vi "TileFPWindows.vi"(5 "Tile Cols":i16=2, 7 "Tile Rows":i16=3, 8 "error in (no error)":errorcluster, 9 "Control Panel Bounds":T1, 10 "Monitor Bounds":T1, 11 "Number of channels":i32) -> (0 "error out":errorcluster, 1 "Not Enough Tiles":bool, 2 "Plot Bounds":T2(array[cluster]))   [LabVIEW 2015]
uses:
  <vilib>/Utility/miscctls.llb/LVRectTypeDef.ctl
panel:
  out "Numeric":i32=1
  out "Numeric 2":i32=1
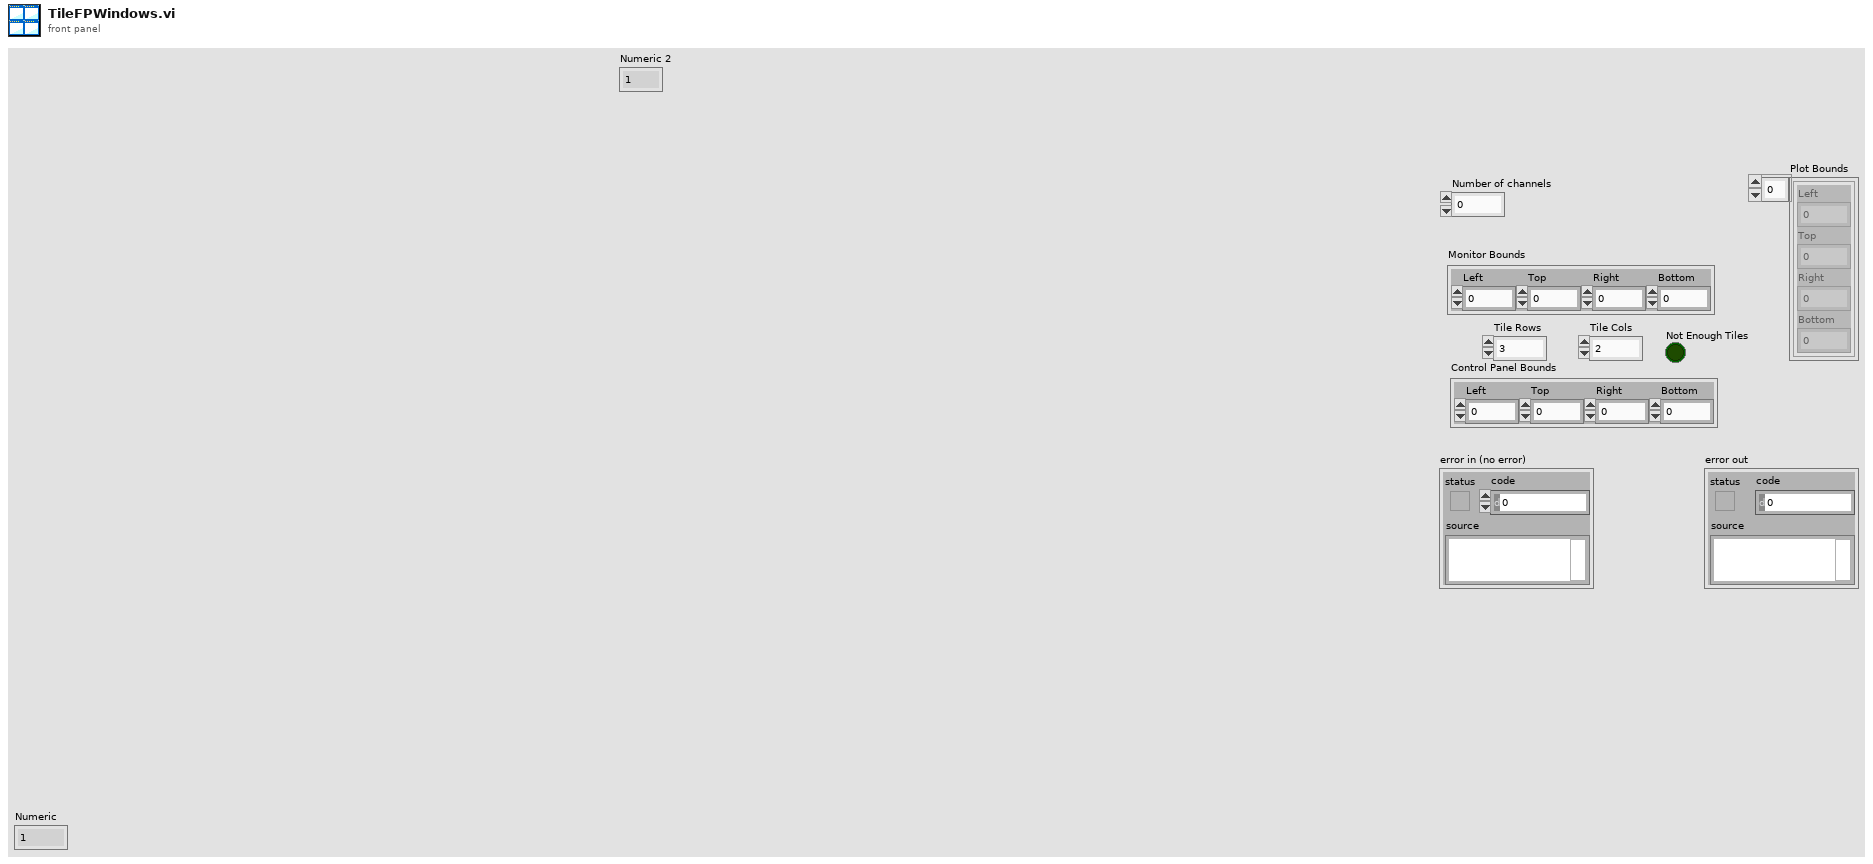
[diagram p1: front panel]
types:
  T1 = typedef "LVRectTypeDef.ctl" = cluster{"Left":i16, "Top":i16, "Right":i16, "Bottom":i16}
  T2 = cluster{"Left":i16, "Top":i16, "Right":i16, "Bottom":i16}[]
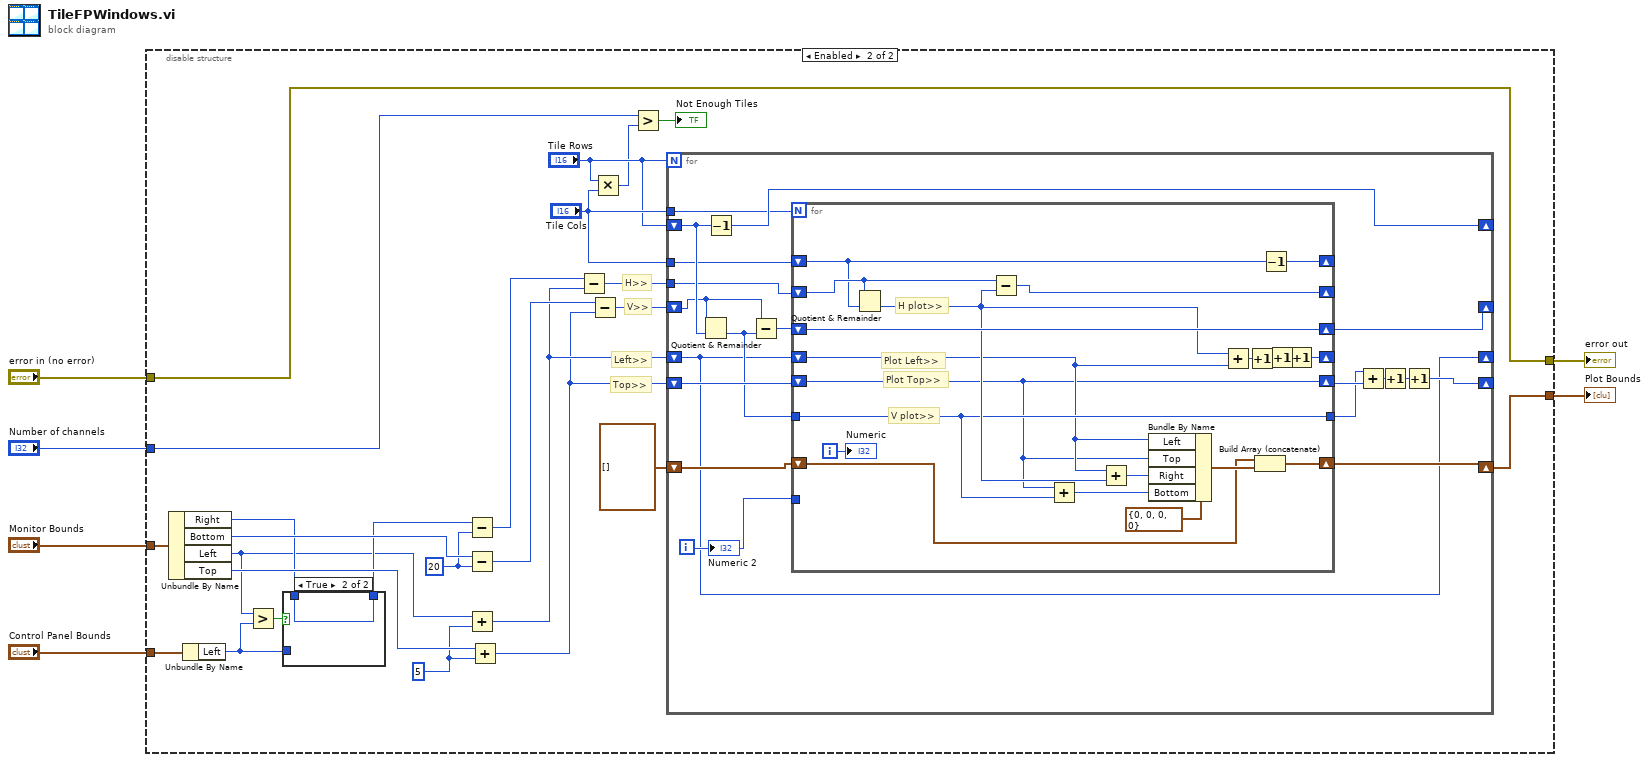
[diagram p0: block diagram]
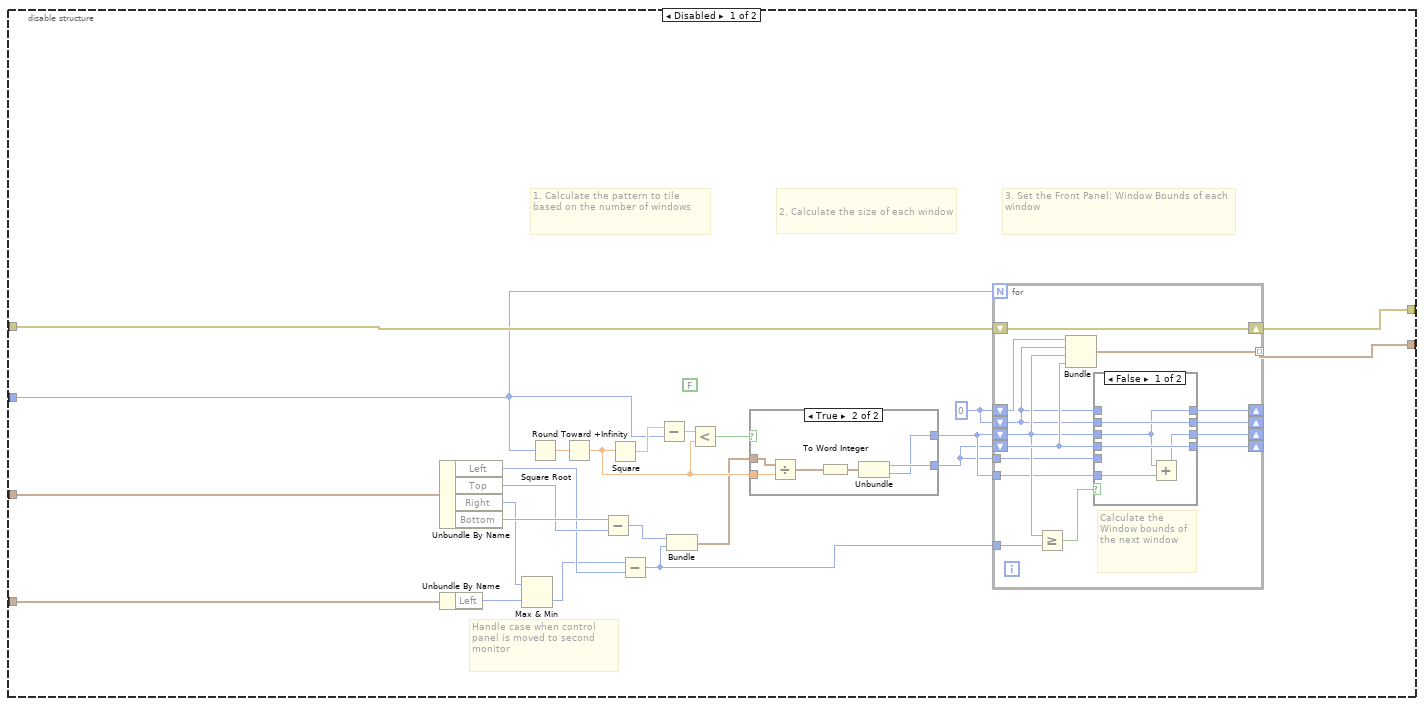
[diagram p2: hidden frame]
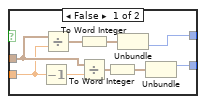
[diagram p3: hidden frame]
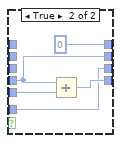
[diagram p4: hidden frame]
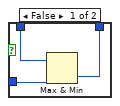
[diagram p5: hidden frame]
diagram:
  n1 = disable-structure shown="Enabled" {
    disable-tunnel: [w29 w85] -> w6
    disable-tunnel: "error in (no error)" -> [w28 w76]
    disable-tunnel: [w27 w76] -> w4
    disable-tunnel: "Control Panel Bounds" -> [w19 w79]
    disable-tunnel: "Monitor Bounds" -> [w18 w93]
    disable-tunnel: "Number of channels" -> [w11 w81]
    frame Disabled {
      (unwired) FALSE
      w26 = i16 0
      # "Handle case when control panel is moved to second monitor"
      # "3. Set the Front Panel: Window Bounds of each window"
      # "2. Calculate the size of each window"
      # "1. Calculate the pattern to tile based on the number of windows"
      n2 = Unbundle By Name(w18) -> ("Left"=w15:i16, "Top"=w16:i16, "Right"=w10:i16, "Bottom"=w17:i16)
      n3 = Unbundle By Name(w19) -> ("Left"=w9:i16)
      n4 = Max & Min(x=w10, y=w9) -> (min(x,y)=w8:i16)  [unwired: 1 out]
      n5 = Square Root(x=w11) -> (sqrt(x)=w25:dbl)
      n6 = Round Toward +Infinity(x=w25) -> (ceil(x): smallest int >= x=w20:dbl)
      n7 = Subtract(x=w17, y=w16) -> (x-y=w14:i16)
      n8 = Square(x=w20) -> (x^2=w24:dbl)
      n9 = Subtract(x=w8, y=w15) -> (x-y=w12:i16)
      n10 = Subtract(x=w24, y=w11) -> (x-y=w23:dbl)
      n11 = Bundle(w14, w12) -> (w13:cluster{i16, i16})  [unwired: 1 in]
      n12 = Less?(x=w23, y=w20) -> (x < y?=w7:bool)
      n13 = case shown="True" w7 {
        tunnel: w13 -> [w33 w42]
        tunnel: [w36 w40] -> w22
        tunnel: [w30 w41] -> w21
        tunnel: w20 -> [w32 w39]
        frame False {
          n14 = Decrement(x=w32) -> (x-1=w31:dbl)
          n15 = Divide(x=w33, y=w32) -> (x/y=w38:cluster{dbl, dbl})
          n16 = To Word Integer(number=w38) -> (16bit integer=w37:cluster{i16, i16})
          n17 = Divide(x=w33, y=w31) -> (x/y=w34:cluster{dbl, dbl})
          n18 = To Word Integer(number=w34) -> (16bit integer=w35:cluster{i16, i16})
          n19 = Unbundle(w37) -> (w36:i16)  [unwired: 1 out]
          n20 = Unbundle(w35) -> (w30:i16)  [unwired: 1 out]
        }
        frame True {
          n21 = Divide(x=w42, y=w39) -> (x/y=w44:cluster{dbl, dbl})
          n22 = To Word Integer(number=w44) -> (16bit integer=w43:cluster{i16, i16})
          n23 = Unbundle(w43) -> (w41:i16, w40:i16)
        }
      }
      n24 = for {
        N: w11 -> [_]
        shift-right: [w50] -> _
        shift-left: w22 -> [w54]
        shift-right: [w51] -> _
        shift-left: w21 -> [w55]
        shift-right: [w52] -> _
        shift-left: w26 -> [w49]
        shift-right: [w53] -> _
        shift-left: w26 -> [w58]
        tunnel: w12 -> [w57]
        tunnel: w21 -> [w48]
        tunnel: w22 -> [w47]
        shift-right: [w46] -> w27
        shift-left: w28 -> [w46]
        tunnel: [w45] -> w29 mode=indexing
        # "Calculate the Window bounds of the next window"
        n25 = Greater Or Equal?(x=w54, y=w57) -> (x >= y?=w56:bool)
        n26 = Bundle(w58, w49, w54, w55) -> (w45:cluster{i16, i16, i16, i16})  [unwired: 1 in]
        n27 = case shown="False" w56 {
          tunnel: w55 -> [w62 w67]
          tunnel: w54 -> [w61 _]
          tunnel: w49 -> [w63 _]
          tunnel: w49 -> [_ _]
          tunnel: [w61 i16 0 ("V")] -> w53
          tunnel: [w63 w67] -> w52
          tunnel: [w62 w66] -> w51
          tunnel: [w60 w64] -> w50
          tunnel: w48 -> [_ w65]
          tunnel: w47 -> [w59 w64]
          frame False {
            n28 = Add(x=w61, y=w59) -> (x+y=w60:i16)
          }
          frame True {
            n29 = Add(x=w67, y=w65) -> (x+y=w66:i16)
          }
        }
      }
    }
    frame Enabled {
      w89 = i16 5 ("y")
      w91 = i16 20 ("y")
      # "Top>>"
      # "V>>"
      # "H>>"
      # "Left>>"
      n30 = Unbundle By Name(w93) -> ("Right"=w78:i16, "Bottom"=w92:i16, "Left"=w71:i16, "Top"=w90:i16)
      n31 = Unbundle By Name(w79) -> ("Left"=w70:i16)
      n32 = Greater?(x=w71, y=w70) -> (0:w69:bool)
      n33 = case shown="True" w69 {
        tunnel: w78 -> [w96 w97]
        tunnel: [w95 w97] -> w77
        tunnel: w70 -> [w94 _]
        frame False {
          n34 = Max & Min(x=w96, y=w94) -> (min(x,y)=w95:i16)  [unwired: 1 out]
        }
        frame True {
        }
      }
      n35 = Subtract(x=w77, y=w91) -> (x-y=w88:i16)
      n36 = Subtract(x=w92, y=w91) -> (x-y=w87:i16)
      n37 = Add(x=w71, y=w89) -> (x+y=w74:i16)
      n38 = Add(x=w90, y=w89) -> (x+y=w72:i16)
      n39 = Subtract(x=w88, y=w74) -> (x-y=w75:i16)
      n40 = Subtract(x=w87, y=w72) -> (x-y=w73:i16)
      n41 = Multiply(x="Tile Rows", y="Tile Cols") -> (x*y=w82:i16)
      n42 = Greater?(x=w81, y=w82) -> (0:→"Not Enough Tiles":bool)
      n43 = for {
        N: "Tile Rows" -> [_]
        shift-right: [w107] -> _
        shift-left: w73 -> [w110]
        shift-right: [w98] -> _
        shift-left: w74 -> [w98]
        shift-right: [w104] -> _
        shift-left: w72 -> [w115]
        shift-right: [w106] -> _
        shift-left: "Tile Rows" -> [w112]
        tunnel: "Tile Cols" -> [w103]
        tunnel: "Tile Cols" -> [w102]
        tunnel: w75 -> [w101]
        shift-right: [w100] -> w85
        shift-left: T1[] [] -> [w99]
        i -> [w116]
        n44 = Quotient & Remainder(x=w110, y=w112) -> (floor(x/y)=w111:i16)  [unwired: 1 out]
        n45 = Decrement(x=w112) -> (x-1=w106:i16)
        n46 = Subtract(x=w110, y=w111) -> (x-y=w109:i16)
        n47 = for {
          N: w103 -> [_]
          tunnel: w116 -> [_]
          shift-right: [w133] -> _
          shift-left: w101 -> [w134]
          shift-right: [w135] -> w107
          shift-left: w109 -> [w135]
          shift-right: [w128] -> _
          shift-left: w98 -> [w119]
          shift-right: [w117] -> w114
          shift-left: w115 -> [w117]
          shift-right: [w132] -> _
          shift-left: w102 -> [w131]
          tunnel: w111 -> [w124]
          tunnel: [w124] -> w108
          shift-right: [w122] -> w100
          shift-left: w99 -> [w121]
          i -> [w127]
          # "Plot Top>>"
          # "Plot Left>>"
          # "V plot>>"
          # "H plot>>"
          n48 = Quotient & Remainder(x=w134, y=w131) -> (floor(x/y)=w125:i16)  [unwired: 1 out]
          n49 = Subtract(x=w134, y=w125) -> (x-y=w133:i16)
          n50 = Add(x=w117, y=w124) -> (x+y=w118:i16)
          n51 = Add(x=w119, y=w125) -> (x+y=w120:i16)
          n52 = Bundle By Name(cluster=T1 {"Left"=0, "Top"=0, "Right"=0, "Bottom"=0} ("Monitor Bounds"), "Left"=w119, "Top"=w117, "Right"=w120, "Bottom"=w118) -> (w123:T1)
          n53 = Add(x=w125, y=w119) -> (x+y=w136:i16)
          n54 = Increment(x=w136) -> (x+1=w130:i16)
          n55 = Build Array (concatenate)(w121, w123) -> (w122:T1[])
          n56 = Decrement(x=w131) -> (x-1=w132:i16)
          n57 = Increment(x=w130) -> (x+1=w129:i16)
          n58 = Increment(x=w129) -> (x+1=w128:i16)
          "Numeric" <- w127
        }
        n59 = Add(x=w108, y=w114) -> (x+y=w113:i16)
        n60 = Increment(x=w113) -> (x+1=w105:i16)
        n61 = Increment(x=w105) -> (x+1=w104:i16)
        "Numeric 2" <- w116
      }
    }
  }
  "error out" <- w4
  "Plot Bounds" <- w6
